vi "Read Allowable Pairing Distances.vi"(8 "error in (no error)":errorcluster, 11 "E2E configuration in":refnum<class "E2E Tag Exchange configuration.lvclass">) -> (0 "error out":errorcluster, 2 "Allowable Pairing Distances":i32[](array[numeric]), 3 "E2E configuration out":refnum<class "E2E Tag Exchange configuration.lvclass">)   [LabVIEW 2015, in "E2E Tag Exchange configuration.lvclass"]
uses:
  E2E Tag Exchange configuration.lvclass
  E2E Tag Exchange configuration.lvclass/E2E Tag Exchange configuration.ctl
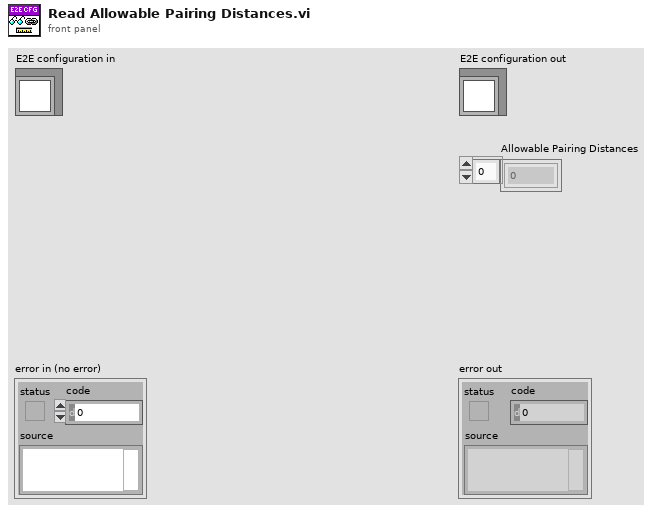
[diagram p1: front panel]
types:
  T1 = typedef "E2E Tag Exchange configuration.lvclass/Runtime Implementation.ctl" = enum16{"RT FIFO", "UDP"}
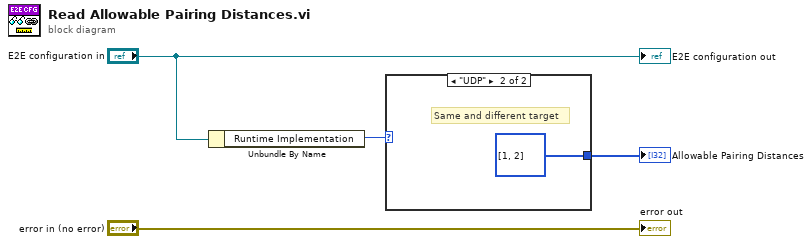
[diagram p0: block diagram]
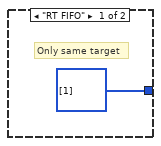
[diagram p2: hidden frame]
diagram:
  n1 = Unbundle By Name("E2E configuration in") -> ("Runtime Implementation"=w2:T1)
  n2 = case shown="\"UDP\"" w2 {
    tunnel: [i32[] [1] i32[] [1, 2]] -> w1
    frame "RT FIFO" {
      # "Only same target"
    }
    frame "UDP" {
      # "Same and different target"
    }
  }
  "Allowable Pairing Distances" <- w1
  "error out" <- "error in (no error)"
  "E2E configuration out" <- "E2E configuration in"
